vi "Control.vi"(6 "Test Duration (Seconds)":i32, 7 "Send File":bool, 8 "error in (no error)":errorcluster, 9 "Stop Test":bool, 10 "Start Test":bool, 11 "Logger in.lvclass":refnum<class "Logger.lvclass">) -> (0 "error out":errorcluster, 2 "Testing":bool, 3 "Logger out.lvclass":refnum<class "Logger.lvclass">)   [LabVIEW 2021, in "Logger.lvclass"]
uses:
  Logger.lvclass
  Logger.lvclass/Logger.ctl
  <vilib>/Skyline/TestMonitor/Shared/typedefs/Status Type.ctl
  <vilib>/Skyline/TestMonitor/Test Result/NI SystemLink Test Result.lvclass/NI SystemLink Test Result.ctl
  <vilib>/Skyline/TestMonitor/Test Result/Write Total Time In Seconds.vi
  <vilib>/Skyline/TestMonitor/Test Result/Write Serial Number.vi
  <vilib>/Skyline/TestMonitor/Test Result/Write Part Number.vi
  <vilib>/Skyline/TestMonitor/Test Result/Update Test Result (Single).vi
  <vilib>/Skyline/TestMonitor/Test Result/Create Test Result (Single).vi
  <vilib>/Skyline/Message/HTTP Wrapper/NI Skyline Message HTTP.lvclass
  <vilib>/Skyline/TestMonitor/Shared/NI SystemLink Test Monitor.lvlib
  <vilib>/Skyline/TestMonitor/Test Result/NI SystemLink Test Result.lvclass
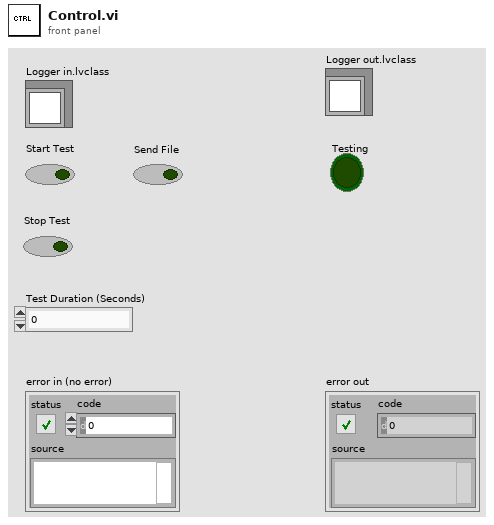
[diagram p1: front panel]
types:
  T1 = typedef "NI SystemLink Test Monitor.lvlib/Status Type.ctl" = enum16{"Failed", "Passed", "Looping", "Skipped", "Custom", "Done", "Running", "Waiting", "Terminated", "Errored", "Timed Out", "None"}
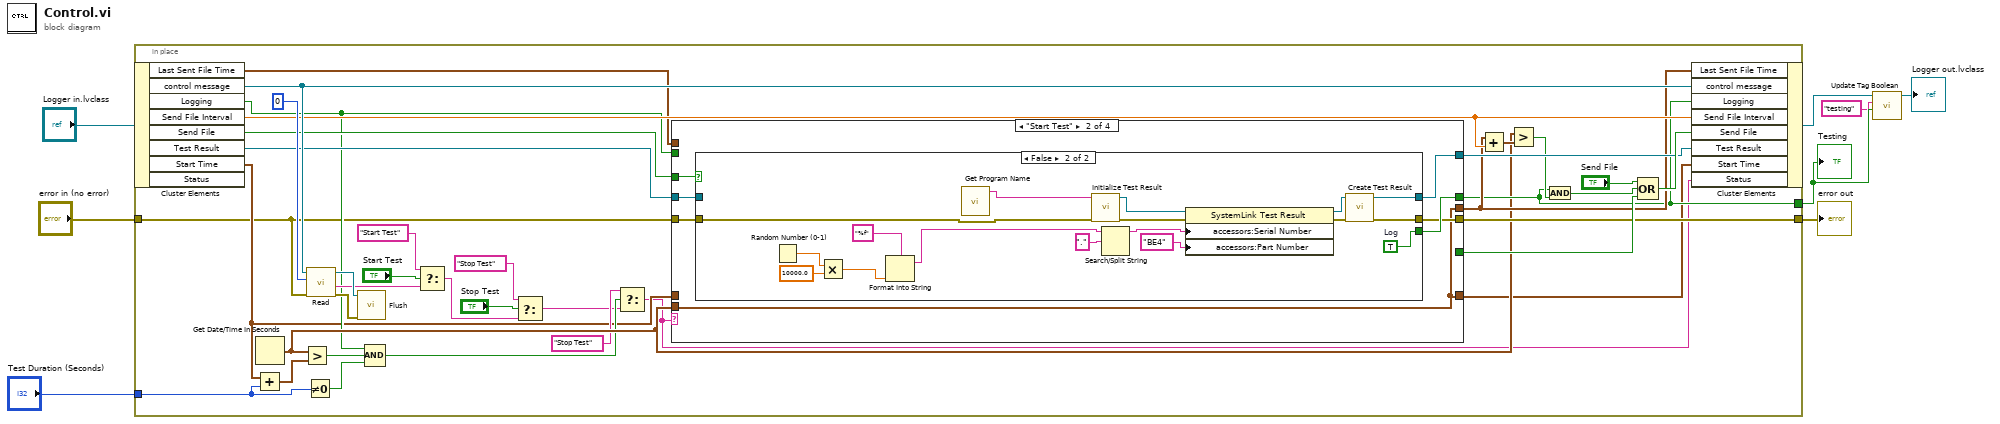
[diagram p0: block diagram]
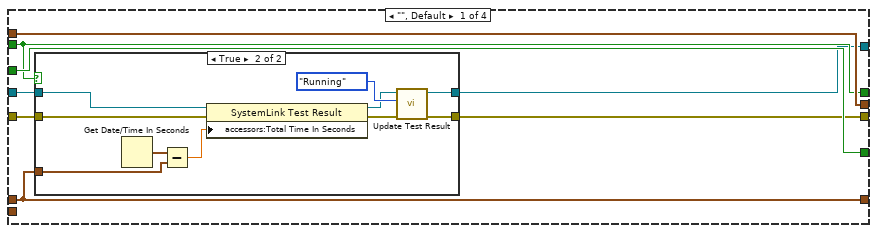
[diagram p2: hidden frame]
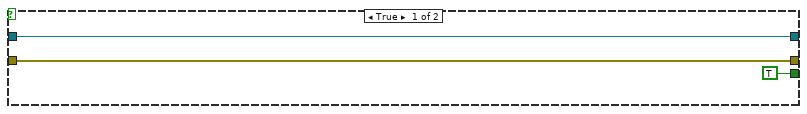
[diagram p4: hidden frame]
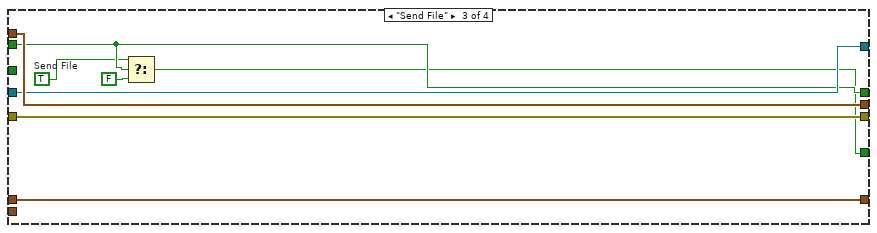
[diagram p5: hidden frame]
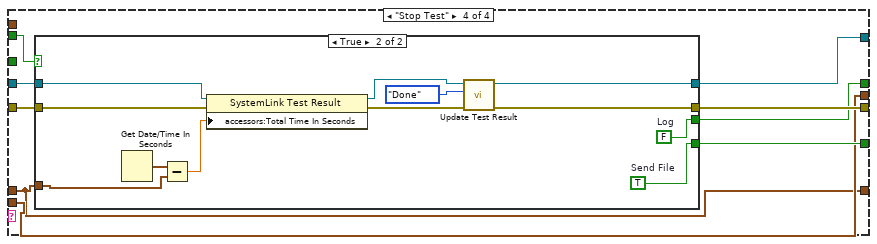
[diagram p6: hidden frame]
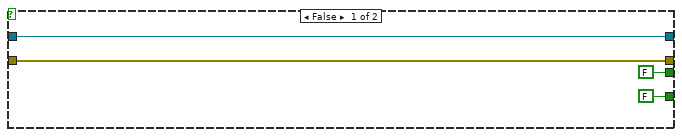
[diagram p7: hidden frame]
diagram:
  n1 = in-place {
    in-place-border: "error in (no error)" -> [w9]
    in-place-border: [w37] -> w6
    in-place-border: [w22] -> w2
    in-place-border: "Test Duration (Seconds)" -> [w12]
    n2 = in-place-cluster #1("Logger in.lvclass") -> ("Last Sent File Time"=w30:timestamp, "control message"=w44:refnum<class "NI Skyline Message HTTP.lvclass">, "Logging"=w16:bool, "Send File Interval"=w39:dbl, "Send File"=w26:bool, "Test Result"=w27:refnum<class "NI SystemLink Test Result.lvclass">, "Start Time"=w13:timestamp)  [unwired: 1 out]
    n3 = Add(x=w13, y=w12) -> (x+y=w20:timestamp)
    n4 = Get Date/Time In Seconds() -> (seconds since 1Jan1904=w21:timestamp)
    n5 = Greater?(x=w21, y=w20) -> (0:w17:bool)
    n6 = Not Equal To 0?(x=w12) -> (x != 0?=w11:bool)
    n7 = call-dynamic "Read.vi"("error in (no error)"=w9, "timeout milliseconds (100)"=0 ("timeout milliseconds"), "sync message session in"=w44) -> ("error out"=w43:errorcluster, "message"=w35:string, "sync message session out"=w42:refnum<class "NI Skyline Message HTTP.lvclass">)  [unwired: 4 in, 2 out]
    n8 = call-dynamic "Flush.vi"("error in (no error)"=w43, "sync message session in"=w42) -> ()  [unwired: 8 in, 2 out]
    n9 = Compound Arithmetic op=AND(w16, w17, w11) -> (w18:bool)
    n10 = Select(t="Start Test", s="Start Test", f=w35) -> (s? t:f=w33:string)
    n11 = Select(t="Stop Test", s="Stop Test", f=w33) -> (s? t:f=w15:string)
    n12 = Select(t="Stop Test", s=w18, f=w15) -> (s? t:f=w10:string)
    n13 = case shown="\"Start Test\"" w10 {
      tunnel: [w51 w72 w96 w106] -> w22
      tunnel: [w52 _ w93 w109] -> w41
      tunnel: w9 -> [w49 w71 w99 w103]
      tunnel: [w46 w70 w99 w108] -> w37
      tunnel: [w53 w68 w100 w105] -> w25
      tunnel: w30 -> [w53 _ w100 _]
      tunnel: [w47 w69 w98 w107] -> w28
      tunnel: w27 -> [w48 w66 w98 w104]
      tunnel: w16 -> [w51 _ w96 w102]
      tunnel: w21 -> [_ w68 _ w105]
      tunnel: w26 -> [w52 w67 _ _]
      tunnel: [w50 w68 w97 w101] -> w14
      tunnel: w13 -> [w50 _ w97 w101]
      frame "", Default {
        n14 = case shown="True" w51 {
          tunnel: [w55 w65] -> w46
          tunnel: [w54 w64] -> w47
          tunnel: w48 -> [w54 w62]
          tunnel: w49 -> [w55 w60]
          tunnel: w50 -> [_ w57]
          frame False {
          }
          frame True {
            n15 = Get Date/Time In Seconds() -> (seconds since 1Jan1904=w58:timestamp)
            n16 = Subtract(x=w58, y=w57) -> (x-y=w56:dbl)
            n17 = property on="Property Node" class="SystemLink Test Result"(reference=w62, error in=w60, "accessors:Total Time In Seconds"=w56) -> (reference out=w61:refnum<class "NI SystemLink Test Result.lvclass">, error out=w59:errorcluster)
            n18 = call-poly <vilib>:"Update Test Result.vi"("error in (no error)"=w59, "status type"=Status_Type."Running", "test result in"=w61) -> ("error out"=w65:errorcluster, "test result out"=w64:refnum<class "NI SystemLink Test Result.lvclass">)  [unwired: 7 in]
          }
        }
      }
      frame "Start Test" {
        n19 = case shown="False" w67 {
          tunnel: [TRUE ("Log") w92] -> w72
          tunnel: w71 -> [w75 w77]
          tunnel: [w75 w90] -> w70
          tunnel: [w74 w89] -> w69
          tunnel: w66 -> [w74 _]
          frame True {
          }
          frame False {
            w92 = TRUE  # Log
            n20 = Random Number (0-1)() -> (number: 0 to 1=w84:dbl)
            n21 = Multiply(x=w84, y=10000.0) -> (x*y=w82:dbl)
            n22 = Format Into String(format string="%f", w82) -> (resulting string=w86:string)  [unwired: 2 in, 1 out]
            n23 = call "Get Program Name.vi"() -> ("String"=w91:string)  [unwired: 11 in]
            n24 = call <vilib>:"Initialize Test Result.vi"("error in (no error)"=w77, "program name"=w91) -> ("error out"=w80:errorcluster, "test result"=w88:refnum<class "NI SystemLink Test Result.lvclass">)  [unwired: 8 in]
            n25 = Search/Split String(string=w86, search string/char (-)=".") -> (substring before match=w76:string)  [unwired: 1 in, 2 out]
            n26 = property class="SystemLink Test Result"(reference=w88, error in=w80, "accessors:Serial Number"=w76, "accessors:Part Number"="BE4" ("Product")) -> (reference out=w81:refnum<class "NI SystemLink Test Result.lvclass">, error out=w79:errorcluster)
            n27 = call-poly <vilib>:"Create Test Result.vi"("error in (no error)"=w79, "test result in"=w81) -> ("error out"=w90:errorcluster, "test result out"=w89:refnum<class "NI SystemLink Test Result.lvclass">)  [unwired: 8 in]
          }
        }
      }
      frame "Send File" {
        w95 = TRUE  # Send File
        n28 = Select(t=w95, s=w96, f=FALSE) -> (s? t:f=w93:bool)
      }
      frame "Stop Test" {
        n29 = case shown="True" w102 {
          tunnel: [FALSE ("Send File") w125] -> w109
          tunnel: [w113 w124] -> w108
          tunnel: [w112 w123] -> w107
          tunnel: [FALSE ("Log") w122] -> w106
          tunnel: w104 -> [w112 w120]
          tunnel: w103 -> [w113 w118]
          tunnel: w101 -> [_ w115]
          frame False {
          }
          frame True {
            w122 = FALSE  # Log
            w125 = TRUE  # Send File
            n30 = Get Date/Time In Seconds() -> (seconds since 1Jan1904=w116:timestamp)
            n31 = Subtract(x=w116, y=w115) -> (x-y=w114:dbl)
            n32 = property on="Property Node" class="SystemLink Test Result"(reference=w120, error in=w118, "accessors:Total Time In Seconds"=w114) -> (reference out=w119:refnum<class "NI SystemLink Test Result.lvclass">, error out=w117:errorcluster)
            n33 = call-poly <vilib>:"Update Test Result.vi"("error in (no error)"=w117, "status type"=Status_Type."Done", "test result in"=w119) -> ("error out"=w124:errorcluster, "test result out"=w123:refnum<class "NI SystemLink Test Result.lvclass">)  [unwired: 7 in]
          }
        }
      }
    }
    n34 = Add(x=w25, y=w39) -> (x+y=w29:timestamp)
    n35 = Greater?(x=w21, y=w29) -> (0:w24:bool)
    n36 = And(x=w22, y=w24) -> (x .and. y?=w23:bool)
    n37 = Compound Arithmetic op=OR("Send File", w23, w41) -> (w40:bool)
    n38 = in-place-cluster #1("Last Sent File Time"=w25, "control message"=w44, "Logging"=w22, "Send File Interval"=w39, "Send File"=w40, "Test Result"=w28, "Start Time"=w14, "Status"=w10) -> (w4:refnum<class "Logger.lvclass">)
  }
  "error out" <- w6
  "Testing" <- w2
  n39 = call "Update Tag Boolean.vi"("Value"=w2, "Tag Path"="testing", "Logger in.lvclass"=w4) -> ("Logger out.lvclass"=→"Logger out.lvclass":refnum<class "Logger.lvclass">)  [unwired: 7 in, 1 out]
